vi "ReadConfig.vi"(8 "error in (no error)":errorcluster) -> (0 "error out":errorcluster, 1 "AcquisitionType":T1, 2 "AnalogOut":T2, 3 "DigitalOut":T3)   [LabVIEW 2020, in "Settings.lvlib"]
uses:
  Settings.lvlib
  Acquisition/DigitalConfig--cluster.ctl
  Acquisition/AnalogConfig--cluster.ctl
  AcqType--enum.ctl
  <vilib>/drjdpowell/SQLite Library/SQL Connection/Open (path).vi
  <vilib>/drjdpowell/SQLite Library/SQL Connection/Open (string).vi
  <vilib>/AdvancedString/Path To Command Line String.vi
  <vilib>/drjdpowell/SQLite Library/SQL Connection/Execute SQL (1D String).vi
  <vilib>/drjdpowell/SQLite Library/SQL Connection/Connection.lvclass
  <vilib>/drjdpowell/SQLite Library/SQLite.lvlib
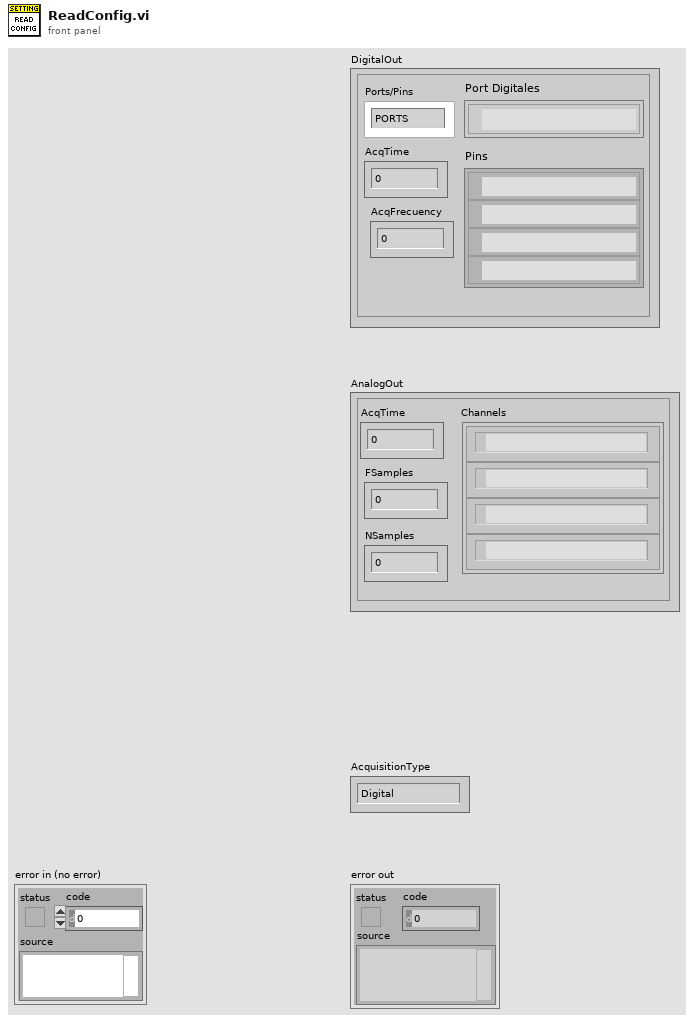
[diagram p1: front panel]
types:
  T1 = typedef "AcqType--enum.ctl" = enum16{"Digital", "Analog"}
  T2 = typedef "AnalogConfig--cluster.ctl" = cluster{"AcqTime":dbl, "FSamples":dbl, "NSamples":dbl, "Channels":tag[]}
  T3 = typedef "DigitalConfig--cluster.ctl" = cluster{"Ports/Pins":enum16{"PORTS", "PINS"}, "AcqTime":dbl, "AcqFrecuency":dbl, "Port Digitales":tag[], "Pins":tag[]}
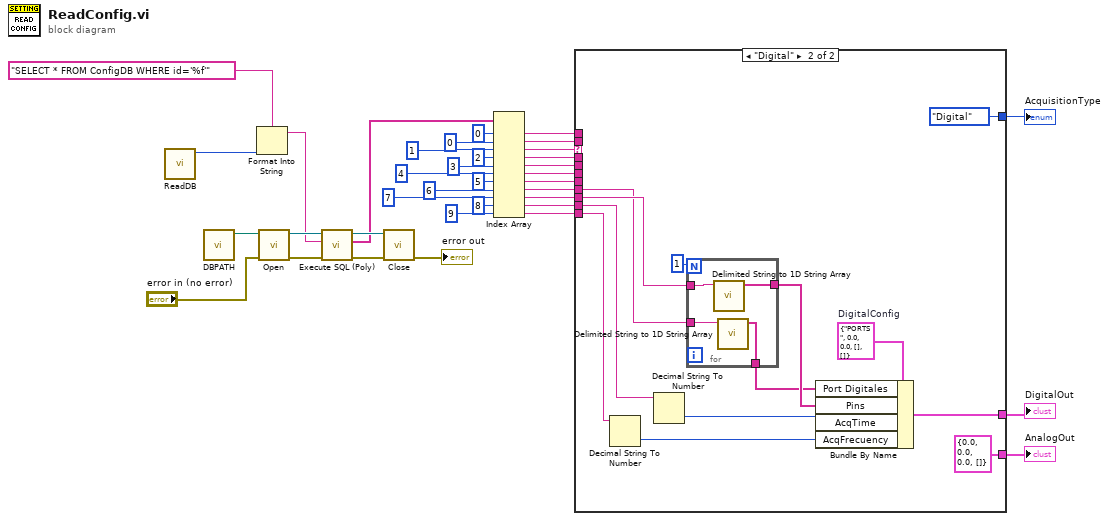
[diagram p0: block diagram]
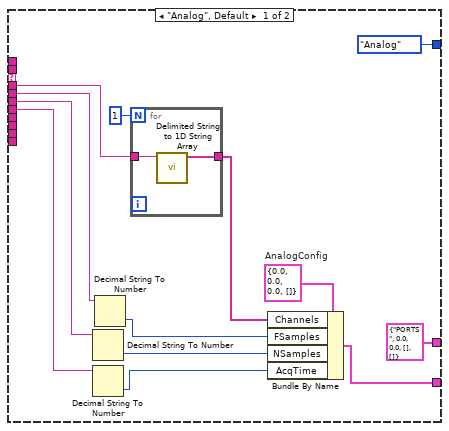
[diagram p2: hidden frame]
diagram:
  n1 = call "ReadDB.vi"() -> ("Max ID"=w28:i32)  [unwired: 8 in, 3 out]
  n2 = call "DBPATH.vi"() -> ("appended path"=w27:path)  [unwired: 11 in]
  n3 = Format Into String(format string="SELECT * FROM ConfigDB WHERE id='%f'" ("SQL"), w28) -> (resulting string=w30:string)  [unwired: 2 in, 1 out]
  n4 = call-poly <vilib>:"Open.vi"("error in (no error)"="error in (no error)", "db file"=w27) -> ("error out"=w36:errorcluster, "SQLite Connection"=w31:refnum<class "Connection.lvclass">)  [unwired: 8 in]
  n5 = call-poly <vilib>:"Execute SQL (Poly).vi"("error in (no error)"=w36, "SQL"=w30, "SQLite Connection in"=w31) -> ("error out"=w35:errorcluster, "Result Set"=w26:string[], "SQLite Connection"=w34:refnum<class "Connection.lvclass">)  [unwired: 5 in, 1 out]
  n6 = call-dynamic "Close.vi"("error in (no error)"=w35, "SQLite Connection in"=w34) -> ("error out"=→"error out":errorcluster)  [unwired: 9 in]
  n7 = Index Array(array=w26, index #1=0 ("index"), index #2=0 ("index"), index #3=1 ("index"), index #4=2 ("index"), index #5=3 ("index"), index #6=4 ("index"), index #7=5 ("index"), index #8=6 ("index"), index #9=7 ("index"), index #10=8 ("index"), index #11=9 ("index")) -> (element #1=w13:string, element #2=w4:string, element #3=w14:string, element #4=w12:string, element #5=w11:string, element #6=w10:string, element #7=w9:string, element #8=w8:string, element #9=w7:string, element #10=w6:string, element #11=w5:string)
  n8 = case shown="\"Digital\"" w14 {
    tunnel: w13 -> [_ _]
    tunnel: w12 -> [w43 _]
    tunnel: w11 -> [w49 _]
    tunnel: w10 -> [w46 _]
    tunnel: w9 -> [w44 _]
    tunnel: w8 -> [_ w57]
    tunnel: w7 -> [_ w59]
    tunnel: w6 -> [_ w60]
    tunnel: w5 -> [_ w63]
    tunnel: w4 -> [_ _]
    tunnel: [T3 {"Ports/Pins"=enum."PORTS", "AcqTime"=0.0, "AcqFrecuency"=0.0, "Port Digitales"=[], "Pins"=[]} ("DigitalConfig") w54] -> w3
    tunnel: [w39 T2 {"AcqTime"=0.0, "FSamples"=0.0, "NSamples"=0.0, "Channels"=[]} ("AnalogConfig")] -> w2
    tunnel: [AcqType--enum."Analog" ("AcquisitionType") AcqType--enum."Digital" ("AcquisitionType")] -> w1
    frame "Analog", Default {
      w40 = T2 {"AcqTime"=0.0, "FSamples"=0.0, "NSamples"=0.0, "Channels"=[]}  # AnalogConfig
      n9 = Decimal String To Number(string=w46) -> (number=w48:i32)  [unwired: 2 in, 1 out]
      n10 = Decimal String To Number(string=w44) -> (number=w45:i32)  [unwired: 2 in, 1 out]
      n11 = Decimal String To Number(string=w49) -> (number=w47:i32)  [unwired: 2 in, 1 out]
      n12 = for {
        N: 1 -> [_]
        tunnel: w43 -> [w50]
        tunnel: [w51] -> w42
        n13 = call <vilib>:"Delimited String to 1D String Array.vi"("delimited string"=w50) -> ("string array"=w51:string[])  [unwired: 10 in]
      }
      n14 = Bundle By Name(cluster=w40, "Channels"=w42, "FSamples"=w47, "NSamples"=w48, "AcqTime"=w45) -> (w39:T2)
    }
    frame "Digital" {
      w55 = T3 {"Ports/Pins"=enum."PORTS", "AcqTime"=0.0, "AcqFrecuency"=0.0, "Port Digitales"=[], "Pins"=[]}  # DigitalConfig
      n15 = Decimal String To Number(string=w63) -> (number=w62:i32)  [unwired: 2 in, 1 out]
      n16 = Decimal String To Number(string=w60) -> (number=w61:i32)  [unwired: 2 in, 1 out]
      n17 = for {
        N: 1 -> [_]
        tunnel: w59 -> [w67]
        tunnel: [w68] -> w58
        tunnel: w57 -> [w66]
        tunnel: [w65] -> w56
        n18 = call <vilib>:"Delimited String to 1D String Array.vi"("delimited string"=w67) -> ("string array"=w68:string[])  [unwired: 10 in]
        n19 = call <vilib>:"Delimited String to 1D String Array.vi"("delimited string"=w66) -> ("string array"=w65:string[])  [unwired: 10 in]
      }
      n20 = Bundle By Name(cluster=w55, "Port Digitales"=w56, "Pins"=w58, "AcqTime"=w61, "AcqFrecuency"=w62) -> (w54:T3)
    }
  }
  "DigitalOut" <- w3
  "AnalogOut" <- w2
  "AcquisitionType" <- w1
